vi "getRawFormat.vi"(0 "Camera in":refnum<class "Camera.lvclass">, 11 "error in (no error)":errorcluster) -> (4 "Camera out":refnum<class "Camera.lvclass">, 6 "rawFormat":enum16{"Word", "Byte"}(ring), 15 "error out":errorcluster)   [LabVIEW 2019, in "Camera.lvclass"]
doc: "Retreive the current raw format of the camera (WORD or BYTE)"
uses:
  Camera.lvclass
  Camera.lvclass/Camera.ctl
  pco.sdk/GeneralCameraControl/GeneralCameraControl.lvlib
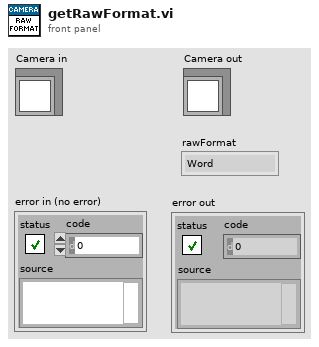
[diagram p1: front panel]
types:
  T1 = enum16{"SETUP_TYPE_SHUTTERMODE", "SETUP_TYPE_PIXELFORMAT", "SETUP_TYPE_SENSOR_DYNRES"}
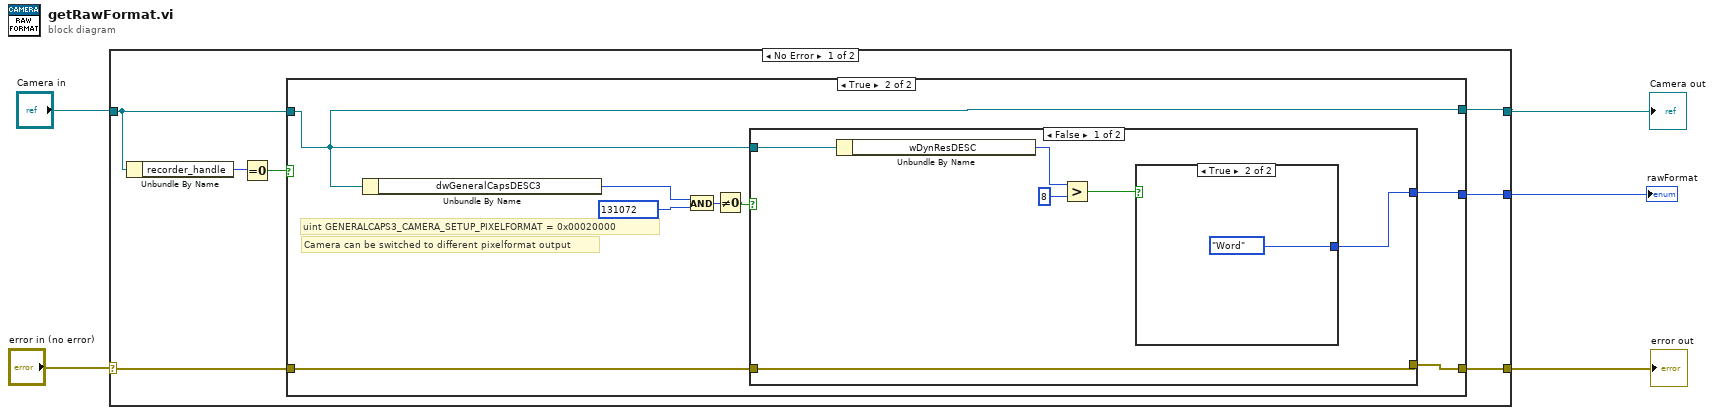
[diagram p0: block diagram]
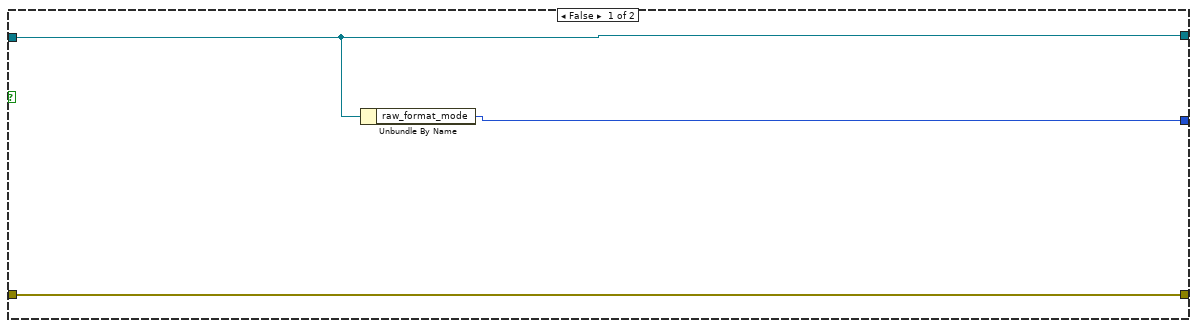
[diagram p2: hidden frame]
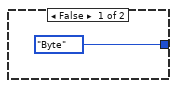
[diagram p3: hidden frame]
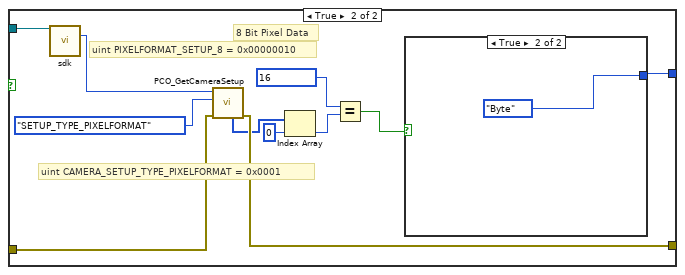
[diagram p4: hidden frame]
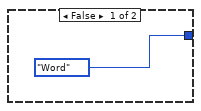
[diagram p5: hidden frame]
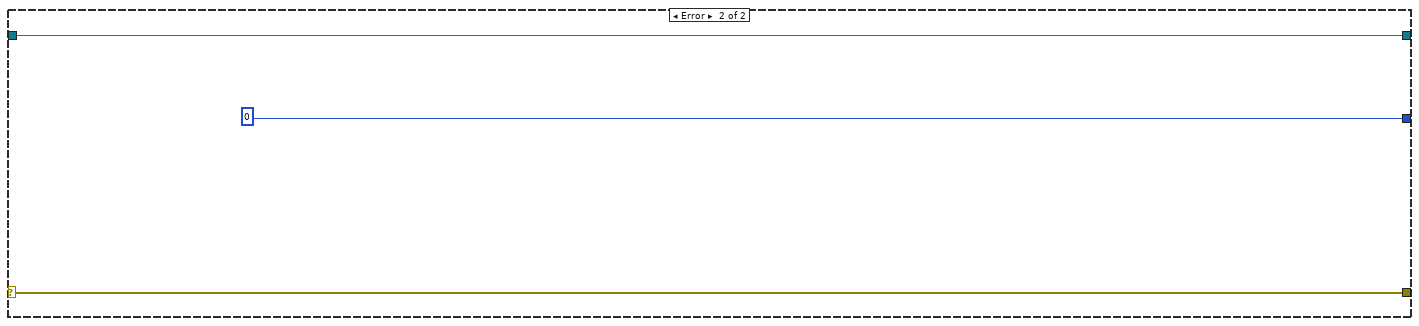
[diagram p6: hidden frame]
diagram:
  n1 = case shown="No Error" "error in (no error)" {
    selector: "error in (no error)" -> [w6 w47]
    tunnel: [w10 w47] -> w3
    tunnel: [w11 w46] -> w4
    tunnel: "Camera in" -> [w9 w46]
    tunnel: [w12 u16 0 ("dwErr")] -> w1
    frame No Error {
      n2 = Unbundle By Name(w9) -> ("recorder_handle"=w8:u64)
      n3 = Equal To 0?(x=w8) -> (x = 0?=w7:bool)
      n4 = case shown="True" w7 {
        tunnel: [w13 w17] -> w12
        tunnel: w9 -> [w14 w18]
        tunnel: [w14 w18] -> w11
        tunnel: w6 -> [w15 w19]
        tunnel: [w15 w16] -> w10
        frame False {
          n5 = Unbundle By Name(w14) -> ("raw_format_mode"=w13:enum16{"Word", "Byte"})
        }
        frame True {
          # "Camera can be switched to different pixelformat output"
          # "uint GENERALCAPS3_CAMERA_SETUP_PIXELFORMAT = 0x00020000"
          n6 = Unbundle By Name(w18) -> ("dwGeneralCapsDESC3"=w23:u32)
          n7 = And(x=w23, y=u32 131072) -> (x .and. y?=w21:u32)
          n8 = Not Equal To 0?(x=w21) -> (x != 0?=w20:bool)
          n9 = case shown="False" w20 {
            tunnel: w19 -> [w24 w42]
            tunnel: [w24 w41] -> w16
            tunnel: w18 -> [w29 w35]
            tunnel: [w25 w33] -> w17
            frame False {
              n10 = Unbundle By Name(w29) -> ("wDynResDESC"=w28:u16)
              n11 = Greater?(x=w28, y=u16 8) -> (0:w26:bool)
              n12 = case shown="True" w26 {
                tunnel: [enum16{"Word", "Byte"}."Byte" ("rawFormat") enum16{"Word", "Byte"}."Word" ("rawFormat")] -> w25
                frame False {
                }
                frame True {
                }
              }
            }
            frame True {
              # "8 Bit Pixel Data"
              # "uint PIXELFORMAT_SETUP_8 = 0x00000010"
              # "uint CAMERA_SETUP_TYPE_PIXELFORMAT = 0x0001"
              n13 = call-dynamic "sdk.vi"("Camera in"=w35) -> ("sdk"=w34:u64)  [unwired: 12 in, 2 out]
              n14 = call "PCO_GetCameraSetup.vi"("error in (no error)"=w42, "wTypeIn"=T1."SETUP_TYPE_PIXELFORMAT", "ph"=w34) -> ("error out"=w41:errorcluster, "dwSetup"=w40:u32[])  [unwired: 4 in, 3 out]
              n15 = Index Array(array=w40, index=0) -> (element=w38:u32)
              n16 = Equal?(x=u32 16, y=w38) -> (x = y?=w36:bool)
              n17 = case shown="True" w36 {
                tunnel: [enum16{"Word", "Byte"}."Word" ("rawFormat") enum16{"Word", "Byte"}."Byte" ("rawFormat")] -> w33
                frame False {
                }
                frame True {
                }
              }
            }
          }
        }
      }
    }
    frame Error {
    }
  }
  "error out" <- w3
  "Camera out" <- w4
  "rawFormat" <- w1
